vi "Galobal variable_TI.vi"() -> ()   [LabVIEW 2015]
panel:
  out "Operator ID":string="OB"
  out "Camera Status":T1
  in  "Shift":T2
  in  "CAM Trigger Right":bool
  in  "CAM Trigger Center":bool
  in  "CAM _Model":i32=14
  in  "Rework Bit":bool
  in  "Camera Trigger":bool
  in  "Tracbility":bool
  out "Pokayoka Status":bool
  in  "NG Count":u8
  out "Shift Change":string
  out "User ID":string="OB"
  in  "RPT Read":bool
  out "Coordinate":string
  out "Camera Ng":bool
  out "Camera Ok":bool
  in  "RPT Write":bool
  in  "Model Trigger":bool
  in  "Camera Write":string
  in  "MIC Barcode Setting":T3={"MIC"="COM1", "MIC Baudrate"=115200.0}
  in  "LOAD NG":bool
  in  "LOad Lvdt data":T4 {"Load Offset" format="%0.03f"; "MaxLoad(N)" format="%0.02f"; "Min Load(N)" format="%0.02f"}
  in  "Load tear bit":bool
  in  "Load Status":string caption="Running Model"
  in  "Camera Result":string caption="Running Model"
  in  "CAM Trigger Left":bool
  in  "Job ID":string caption="Running Model"
  in  "Part Code _Dn":string caption="Running Model"
  in  "Part Code _Up":string caption="Running Model"
  in  "Part Code _Dail LH":string caption="Running Model"
  in  "Part Code _Dail RH":string caption="Running Model"
  in  "MIC BARCODE":string caption="Running Model"
  out "Reset":bool
  out "Emergency":bool
  in  "Load value":dbl format="%0.03f"
  in  "Running Model":string
  in  "Load offset":dbl format="%0.03f"
  in  "Sensor Setting Data":T5
  out "Sensor Data":T6
  in  "NI Comm.Error":bool
  in  "LVDT":dbl format="%0.03f"
  in  "Load Cell":dbl format="%0.03f"
  in  "Digital Output":bool[](array[boolean])
  in  "Auto Exit":bool
  in  "Slid Servo Home bit":bool
  in  "Call Home M2":bool
  in  "Call Home M1":bool
  in  "Barcode Lenght":i32
  in  "Barcode Scan Bit":bool
  in  "Barcode Data":string
  in  "Control Enable":bool
  in  "Stop M1":bool
  in  "Stop M2":bool
  in  "Programlist":string[](array[string])
  in  "STM Done Bit":bool
  in  "Offset_2":dbl
  in  "Offset_1":dbl
  in  "Slop _2":dbl
  in  "Slop_1":dbl
  out "Analoge Input":dbl[](array[numeric])
  out "AI_as DI":bool[](array[boolean])
  out "Manual DO":bool[](array[boolean])
  in  "Manual CMD":bool
  out "File Path":path[](array[path])
  out "Digital input":bool[](array[boolean])
  in  "User Name":string
  in  "Exit":bool
  # "LOad Lvdt data"
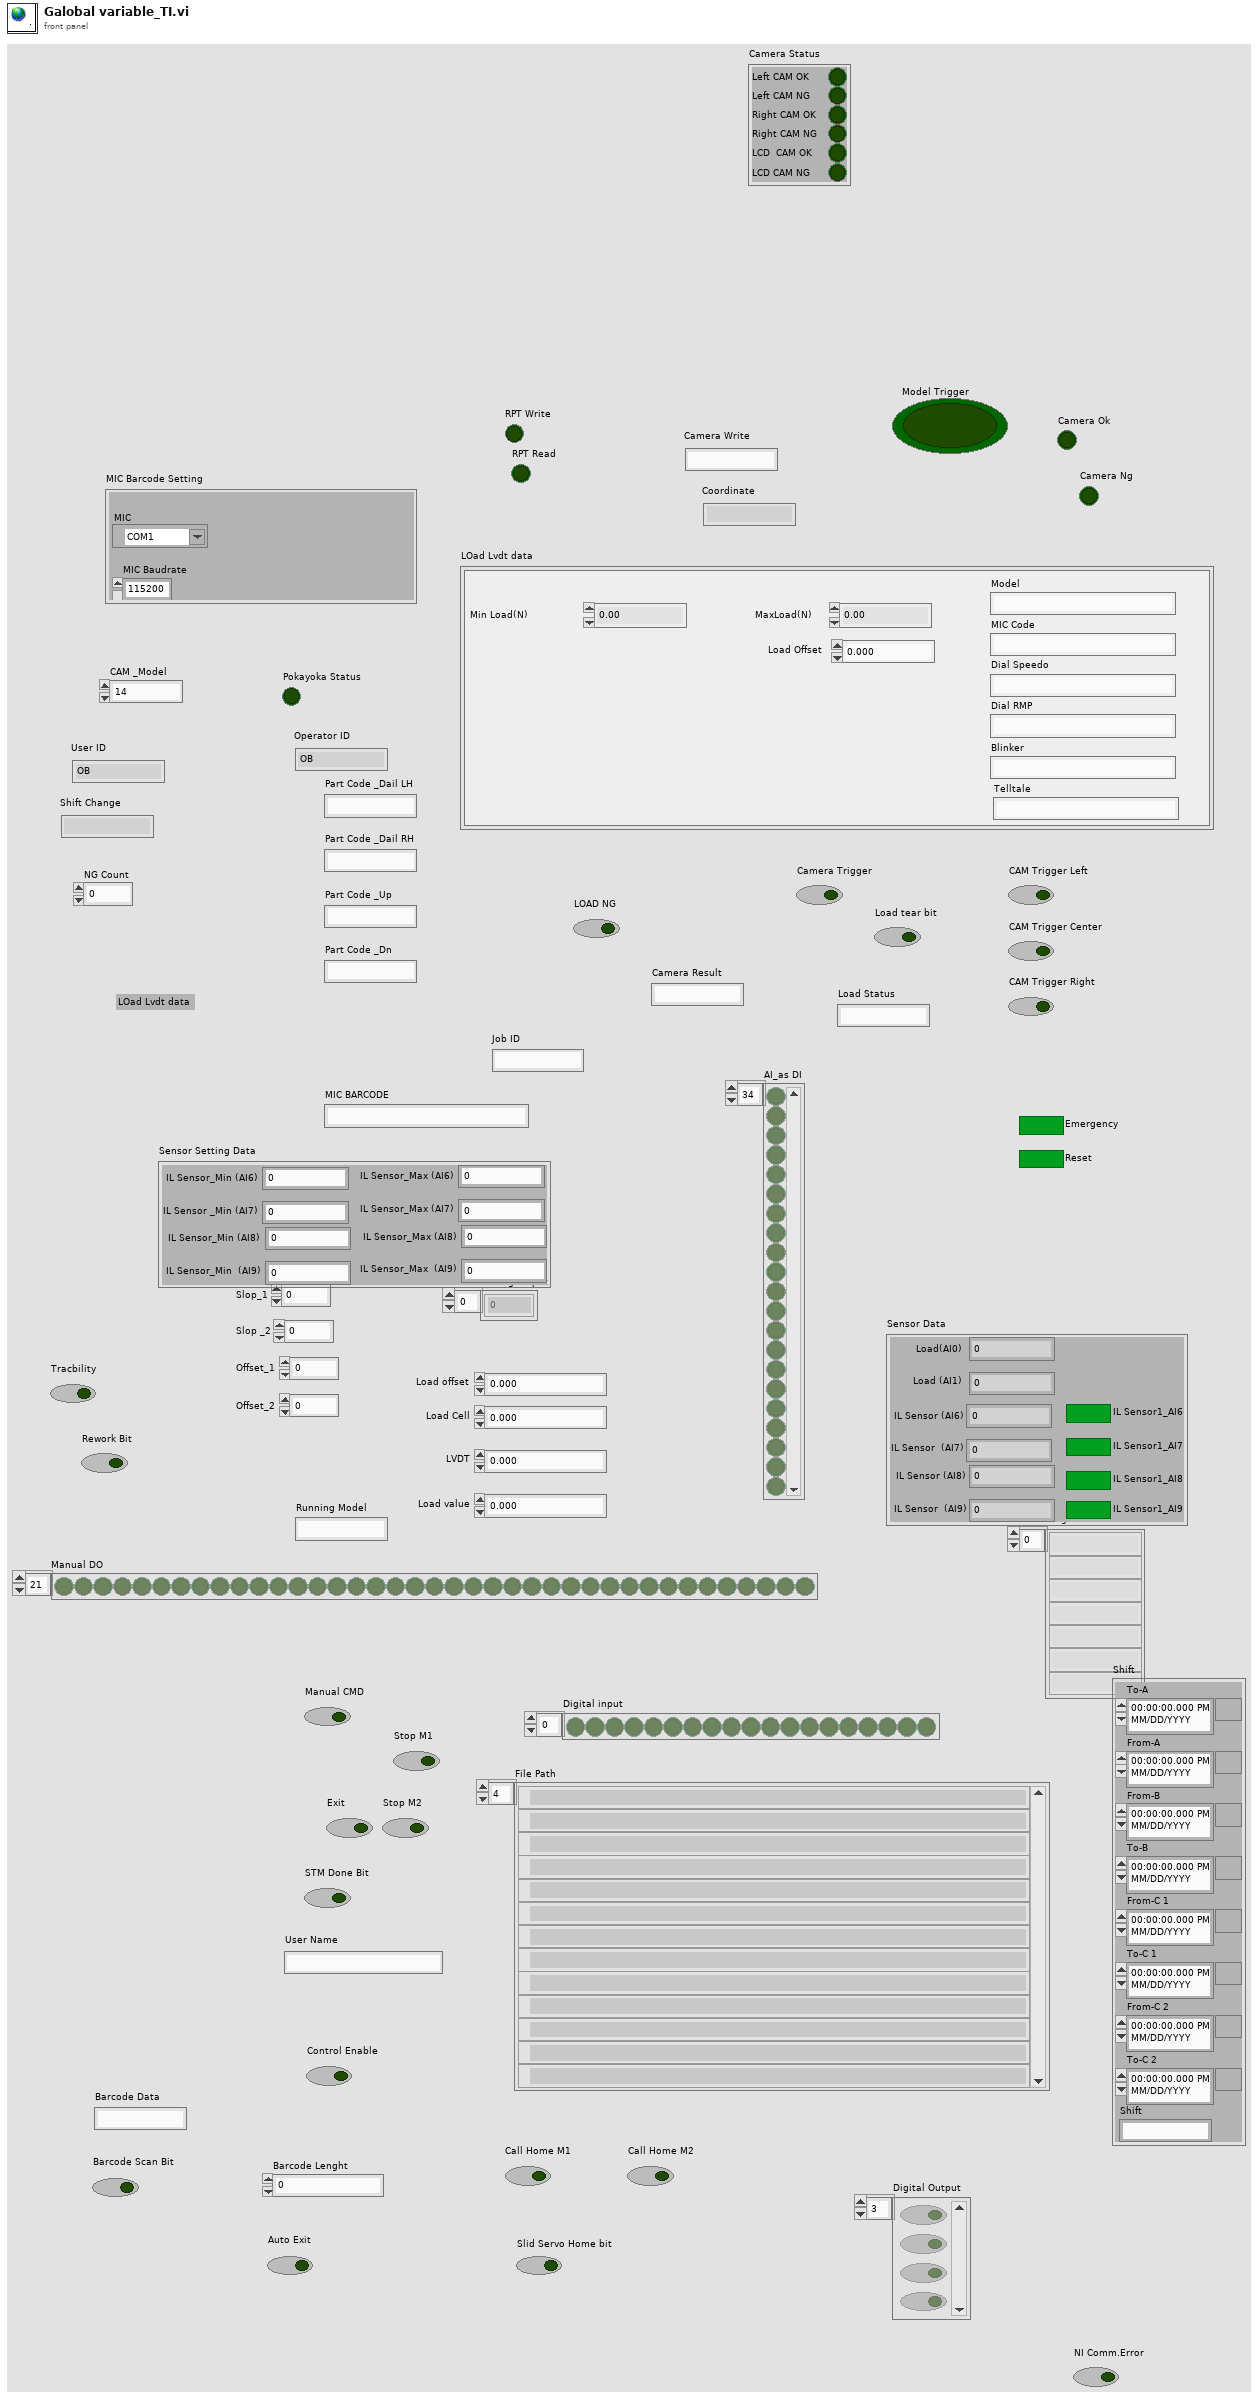
[diagram p1: front panel]
types:
  T1 = cluster{"Left CAM OK":bool, "Left CAM NG":bool, "Right CAM OK":bool, "Right CAM NG":bool, "LCD  CAM OK":bool, "LCD CAM NG ":bool}
  T2 = cluster{"To-A":timestamp, "From-A":timestamp, "From-B":timestamp, "To-B":timestamp, "From-C 1":timestamp, "To-C 1":timestamp, "From-C 2":timestamp, "To-C 2":timestamp, "Shift":string}
  T3 = cluster{"MIC":refnum<visa-resource-name>, "MIC Baudrate":dbl}
  T4 = cluster{"MaxLoad(N) ":dbl, "Min Load(N)":dbl, "Load Offset":dbl, "Model":string, "MIC Code":string, "Dial Speedo":string, "Dial RMP":string, "Blinker":string, "Telltale":string}
  T5 = cluster{"IL Sensor_Max (AI6)":dbl, "IL Sensor_Min (AI6)":dbl, "IL Sensor_Max (AI7)":dbl, "IL Sensor _Min (AI7)":dbl, "IL Sensor_Max (AI8)":dbl, "IL Sensor_Min (AI8)":dbl, "IL Sensor_Max  (AI9)":dbl, "IL Sensor_Min  (AI9)":dbl}
  T6 = cluster{"Load(AI0) ":dbl, "Load (AI1) ":dbl, "IL Sensor (AI6)":dbl, "IL Sensor  (AI7)":dbl, "IL Sensor (AI8)":dbl, "IL Sensor  (AI9)":dbl, "IL Sensor1_AI6":bool, "IL Sensor1_AI7":bool, "IL Sensor1_AI8":bool, "IL Sensor1_AI9":bool}
diagram:
